vi "ApplyConfigInstantly.vi"(8 "error in":errorcluster, 11 "T560Session in":refnum<class "T560Session.lvclass">) -> (0 "error out":errorcluster, 3 "T560Session out":refnum<class "T560Session.lvclass">)   [LabVIEW 2020, in "T560Session.lvclass"]
doc: "Instantly send the channels configuration to the physical device"
uses:
  T560Session.lvclass
  T560Session.lvclass/T560Session.ctl
  T560Channel.lvclass
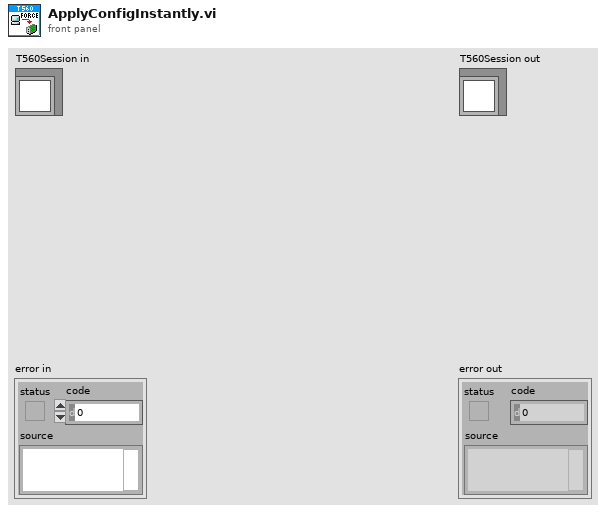
[diagram p1: front panel]
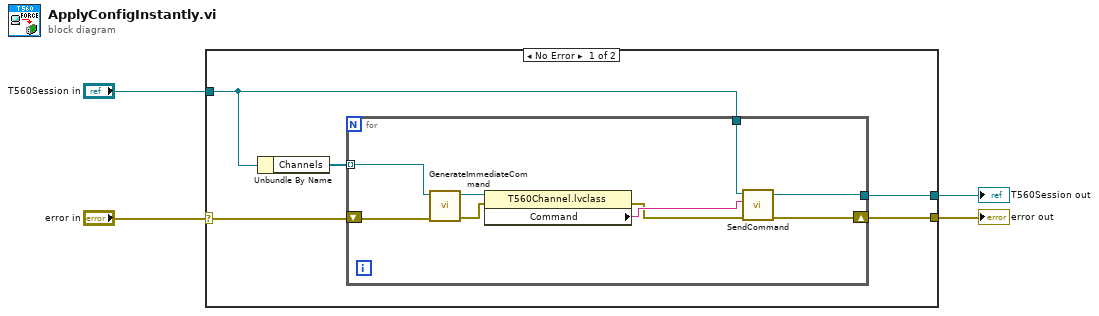
[diagram p0: block diagram]
diagram:
  n1 = case shown="No Error" "error in" {
    selector: "error in" -> [w8 w20]
    tunnel: [w7 w20] -> w3
    tunnel: [w5 w19] -> w1
    tunnel: "T560Session in" -> [w6 w19]
    frame No Error {
      n2 = Unbundle By Name(w6) -> ("Channels"=w9:refnum<class "T560Channel.lvclass">[])
      n3 = for {
        tunnel: w9 -> [w14] mode=indexing
        tunnel: w6 -> [w13]
        shift-right: [w12] -> w7
        shift-left: w8 -> [w18]
        tunnel: [w11] -> w5
        n4 = call-dynamic "GenerateImmediateCommand.vi"("error in"=w18, "T560Object in"=w14) -> ("error out"=w17:errorcluster, "T560Object out"=w10:refnum<class "T560Channel.lvclass">)  [unwired: 8 in]
        n5 = property class="T560Channel.lvclass"(reference=w10, error in=w17) -> (error out=w15:errorcluster, "Command"=w16:string)  [unwired: 1 out]
        n6 = call-dynamic "SendCommand.vi"("error in"=w15, "Command"=w16, "T560Session in"=w13) -> ("error out"=w12:errorcluster, "T560Session out"=w11:refnum<class "T560Session.lvclass">)  [unwired: 6 in, 1 out]
      }
    }
    frame Error {
    }
  }
  "error out" <- w3
  "T560Session out" <- w1
